vi "Set ICommunicate.vi"(10 "ICommunicate":refnum<class "ICommunicate.lvclass">, 11 "Worker in":refnum<class "Communicator Worker.lvclass">) -> (3 "Worker out":refnum<class "Communicator Worker.lvclass">)   [LabVIEW 2019, in "Communicator Worker.lvlib" / "Communicator Worker.lvclass"]
uses:
  Communicator Worker.lvclass
  Interfaces/ICommunicate/ICommunicate.lvclass
  Communicator Worker.lvclass/Communicator Worker.ctl
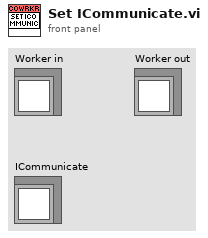
[diagram p1: front panel]
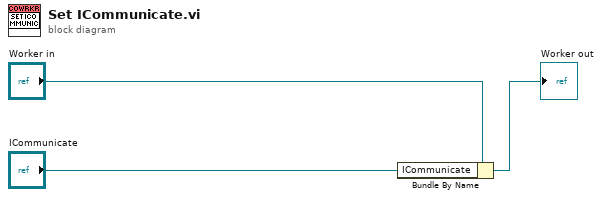
[diagram p0: block diagram]
diagram:
  n1 = Bundle By Name(cluster="Worker in", "ICommunicate"="ICommunicate") -> (→"Worker out":refnum<class "Communicator Worker.lvclass">)
